vi "convertToHtml.vi"(8 "error in (no error)":errorcluster, 10 "HTML File Path":path, 11 "MS-Word in":refnum<class "MS-Word.lvclass">) -> (0 "error out":errorcluster, 3 "MS-Word out":refnum<class "MS-Word.lvclass">)   [LabVIEW 2017, in "LabVIEW NPOI.lvlib" / "MS-Word.lvclass"]
uses:
  MS-Word.lvclass
  MS-Word.lvclass/MS-Word.ctl
  xwpfDocument/xwpfDocument.lvclass/xwpfDocument.ctl
  C:/Users/Neo/Desktop/Dev_Tools_BR/LabVIEW_NPOI/src/lib/NPOI 2.1.1/NPOI.OOXML.dll
  lib/NPOI 2.1.1/NPOI.OOXML.dll
  xwpfDocument/Get Document.Ref.vi
  xwpfDocument/xwpfDocument.lvclass
  Support/File Stream/File Stream.lvlib
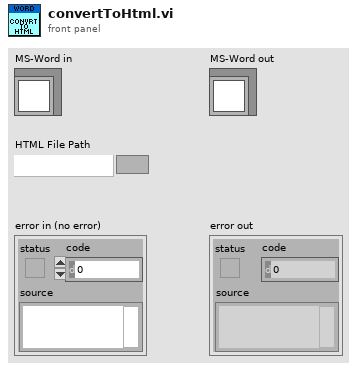
[diagram p1: front panel]
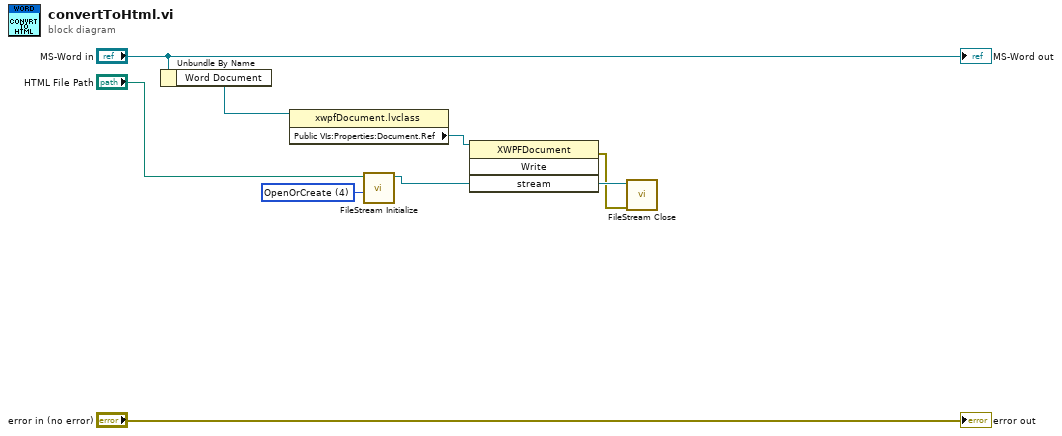
[diagram p0: block diagram]
diagram:
  w1 = 4 items=["CreateNew"=1, "Create"=2, "Open"=3, "OpenOrCreate"=4, "Truncate"=5, "Append"=6] ("mode")
  n1 = Unbundle By Name("MS-Word in") -> ("Word Document"=w6:refnum<class "xwpfDocument.lvclass">)
  n2 = property class="xwpfDocument.lvclass"(reference=w6) -> ("Public VIs:Properties:Document.Ref"=w5:refnum<k24>)  [unwired: 1 in, 2 out]
  n3 = call "FileStream Initialize.vi"("mode"=w1, "path"="HTML File Path") -> ("new reference"=w4:refnum<k24>)  [unwired: 8 in, 1 out]
  n4 = invoke class="XWPFDocument" method="Write"(reference=w5, "stream"=w4) -> (error out=w3:errorcluster)  [unwired: 2 in, 3 out]
  n5 = call "FileStream Close.vi"("error in (no error)"=w3, "reference"=w4) -> ()  [unwired: 9 in, 1 out]
  "error out" <- "error in (no error)"
  "MS-Word out" <- "MS-Word in"
